vi "Moving_FFID_Analysis.vi"() -> (5 "Plug in titles":string[](array[string]), 7 "Plug in values":string[](array[string]))   [LabVIEW 2010]
uses:
  Globals/Plug_in_data_global.vi
  Globals/Meas_global.vi
  <vilib>/Analysis/NI_AALPro.lvlib
panel:
  in  "Downsize points":i32
  out "Rejected Blocks":i32
  in  "Traverse Speed Factor":string
  in  "Number of Samples":string
  out "Pdf":cluster{"Axis":dbl[], dbl[]}(graph)
  in  "Histogram Time":dbl format="%.2f"
  out "Current Block No":i32
  in  "Save averaged traces?":bool
  out "No of Valid Blocks":dbl
  out "FFID Trace Even":cluster{dbl, dbl, dbl[]}(graph)
  out "FFID Trace odd":cluster{dbl, dbl, dbl[]}(graph)
  out "Source On":i32
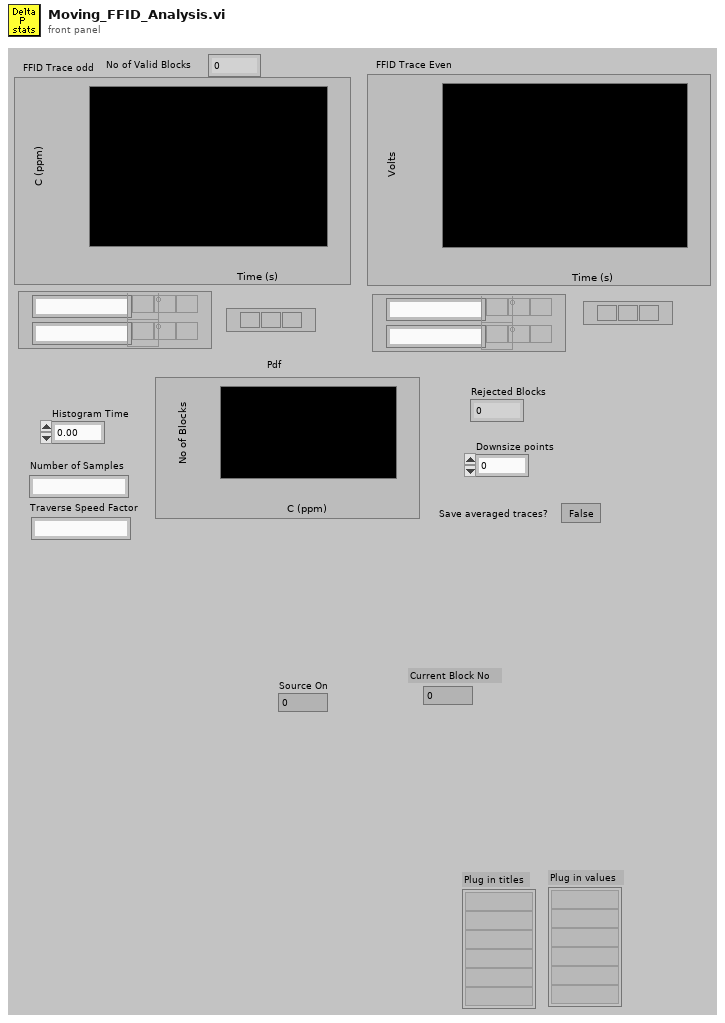
[diagram p1: front panel]
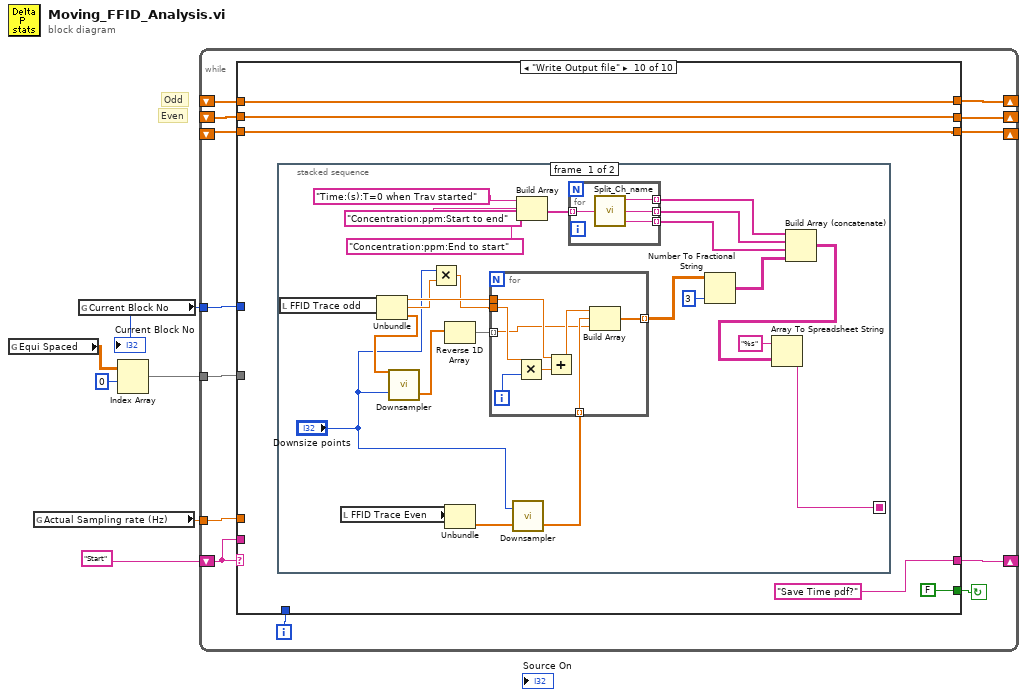
[diagram p0: block diagram]
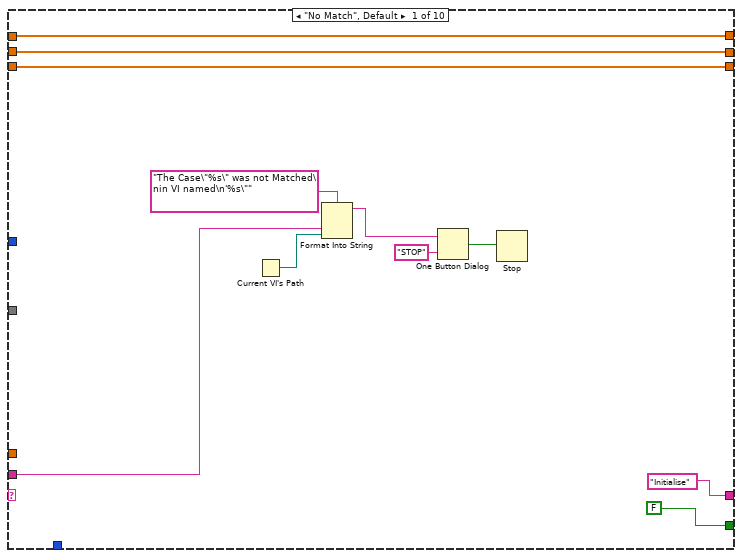
[diagram p2: hidden frame]
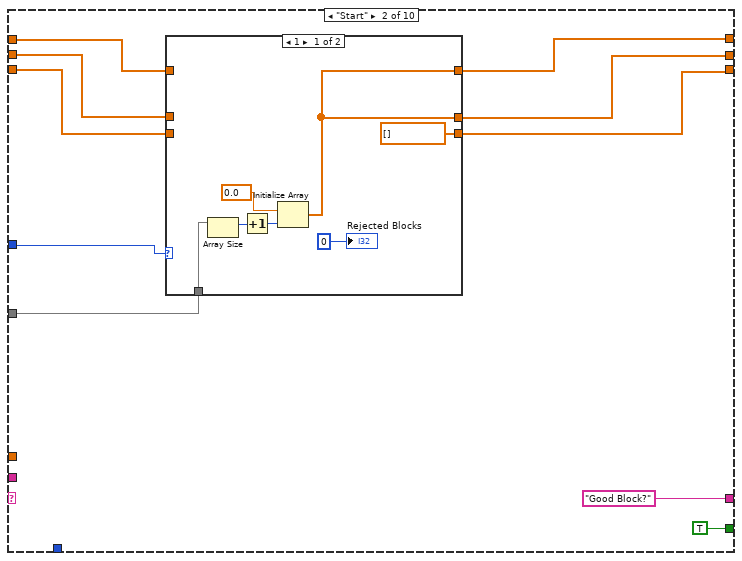
[diagram p3: hidden frame]
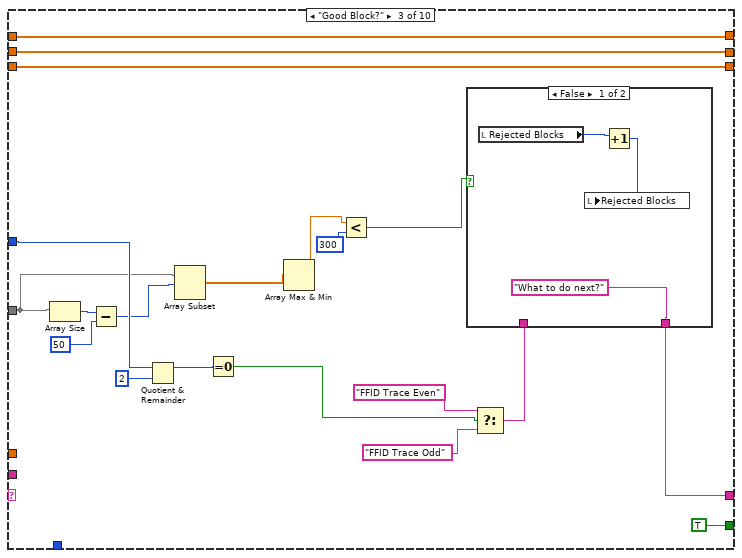
[diagram p5: hidden frame]
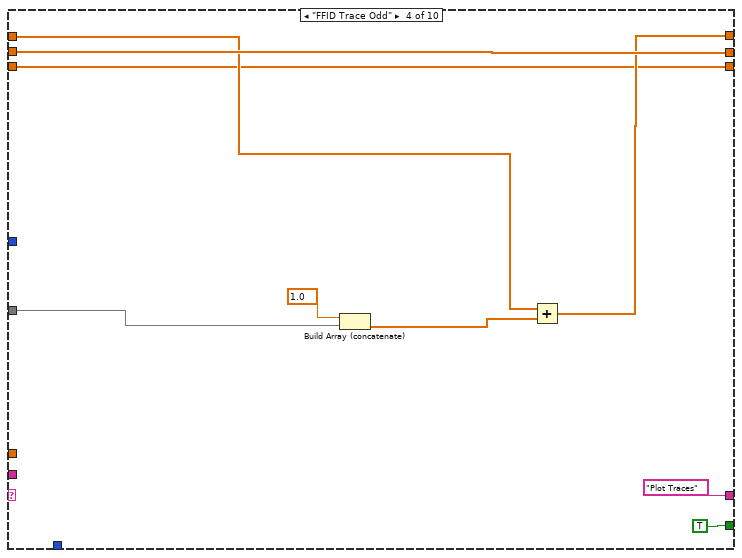
[diagram p7: hidden frame]
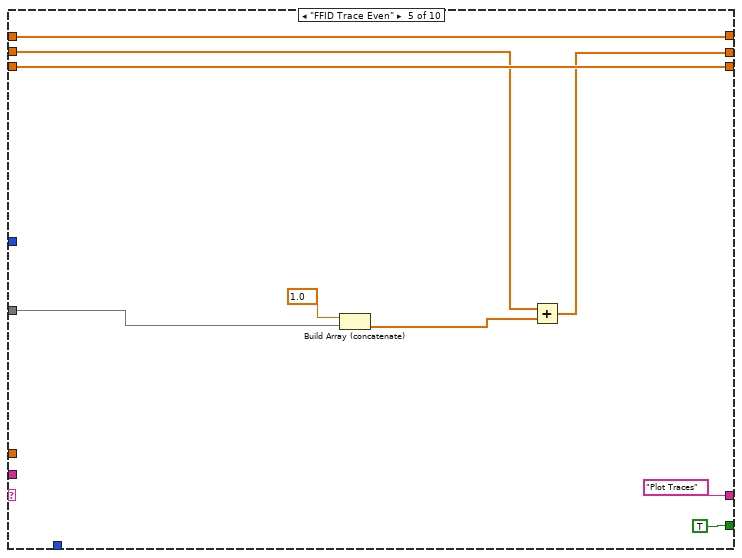
[diagram p8: hidden frame]
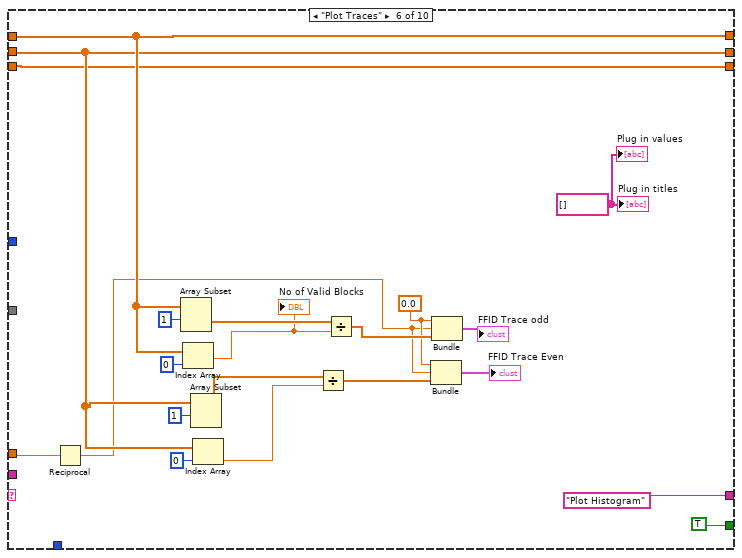
[diagram p9: hidden frame]
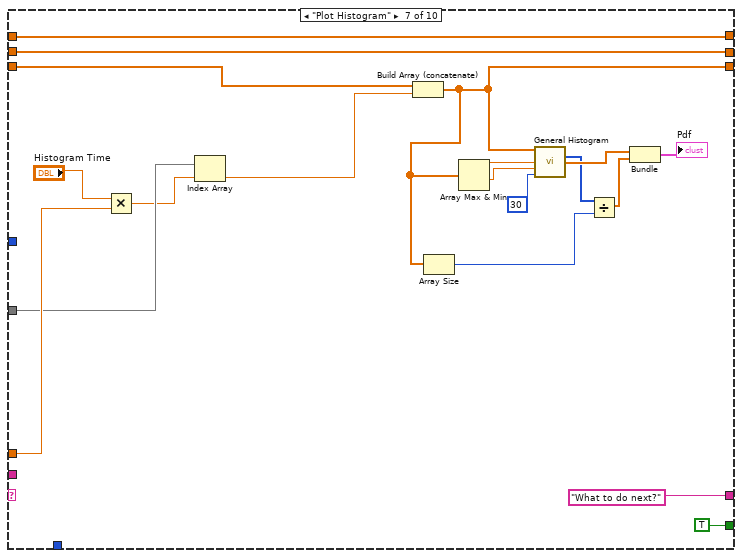
[diagram p10: hidden frame]
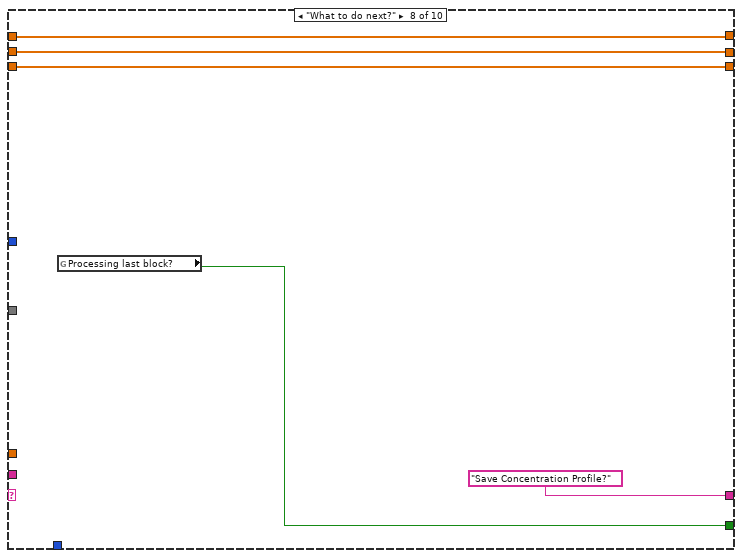
[diagram p11: hidden frame]
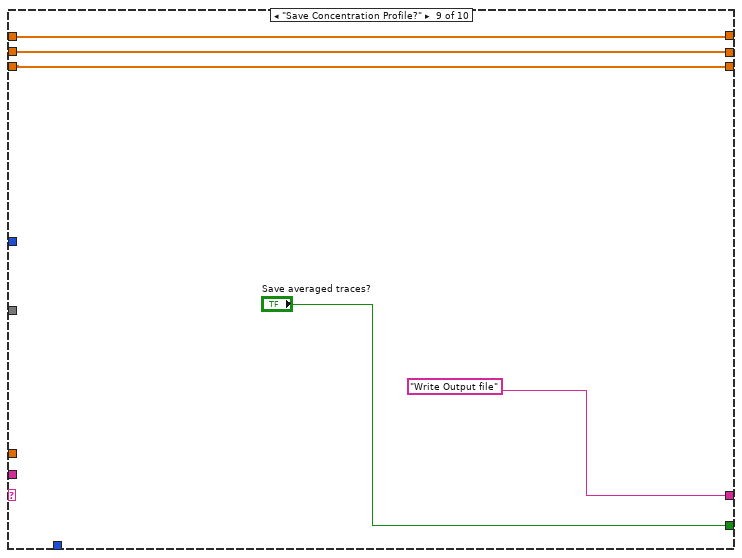
[diagram p12: hidden frame]
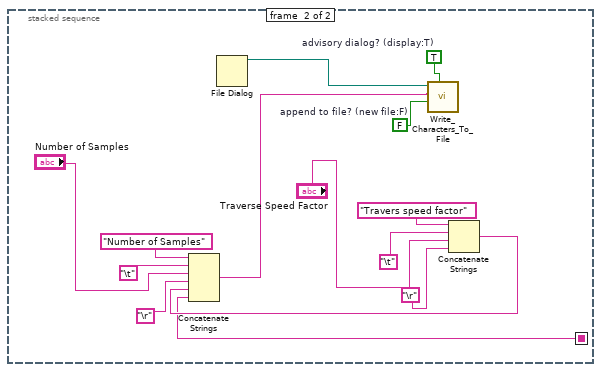
[diagram p13: hidden frame]
diagram:
  # "Even"
  # "Odd"
  n1 = global read "Plug_in_data_global.vi" "Equi Spaced"() -> (w1:dbl[][])
  n2 = global read "Meas_global.vi" "Actual Sampling rate (Hz)"() -> (w3:dbl)
  n3 = global read "Meas_global.vi" "Current Block No"() -> (w2:i32)
  "Current Block No" <- w2
  n4 = Index Array(array=w1, index (row)=0) -> (element=w4:dbl[])  [unwired: 1 in]
  n5 = while {
    shift-left: "Start" -> [w17]
    shift-right: [w18] -> _
    shift-right: [w16] -> _
    shift-left: _ -> [w13]
    shift-right: [w15] -> _
    shift-left: _ -> [w14]
    tunnel: w4 -> [w12]
    tunnel: w3 -> [w11]
    tunnel: w2 -> [w10]
    shift-right: [w7] -> _
    shift-left: _ -> [w8]
    i -> [w9]
    stop <- w19 continue-if-true
    n6 = case shown="\"Write Output file\"" w17 {
      tunnel: [FALSE TRUE ("Processing last block?") TRUE ("Processing last block?") TRUE ("Processing last block?") TRUE ("Processing last block?") TRUE ("Processing last block?") TRUE ("Processing last block?") w133 "Save averaged traces?" FALSE ("Processing last block?")] -> w19
      tunnel: ["Initialise" "Good Block?" w52 "Plot Traces" "Plot Traces" "Plot Histogram" ("f") "What to do next?" ("f") "Save Concentration Profile?" ("t") "Write Output file" "Save Time pdf?"] -> w18
      tunnel: w17 -> [w25 _ _ _ _ _ _ _ _ _]
      tunnel: [w22 w39 w70 w80 w86 w111 w132 w137 w142 w147] -> w16
      tunnel: [w21 w37 w69 w81 w84 w107 w131 w136 w138 w146] -> w15
      tunnel: w14 -> [w21 w36 w69 w81 w85 w107 w131 w136 w138 w146]
      tunnel: w13 -> [w22 w38 w70 w79 w86 w111 w132 w137 w142 w147]
      tunnel: w12 -> [_ w35 w60 w75 w87 _ w128 _ _ _]
      tunnel: w11 -> [_ _ _ _ _ w103 w129 _ _ _]
      tunnel: w10 -> [_ w34 w65 _ _ _ _ _ _ _]
      tunnel: w9 -> [_ _ _ _ _ _ _ _ _ _]
      tunnel: w8 -> [w20 w32 w68 w76 w88 w98 w125 w135 w141 w143]
      tunnel: [w20 w33 w68 w76 w88 w98 w117 w135 w141 w143] -> w7
      frame "No Match", Default {
        n7 = Current VI's Path() -> (path=w24:path)
        n8 = Format Into String(format string="The Case\"%s\" was not Matched\nin VI named\n'%s\"" ("Format String"), w25, w24) -> (resulting string=w28:string)  [unwired: 2 in, 1 out]
        n9 = One Button Dialog(message=w28, button name ("OK")="STOP") -> (true=w26:bool)
        n10 = Stop(stop? (T)=w26) -> ()
      }
      frame "Start" {
        n11 = case shown="1" w34 {
          tunnel: [w44 w50] -> w39
          tunnel: w38 -> [_ w50]
          tunnel: [w44 w49] -> w37
          tunnel: w36 -> [_ w49]
          tunnel: w35 -> [w47 _]
          tunnel: [dbl[] [] w48] -> w33
          tunnel: w32 -> [_ w48]
          frame 1 {
            n12 = Array Size(array=w47) -> (size(s)=w46:i32)
            n13 = Increment(x=w46) -> (x+1=w42:i32)
            n14 = Initialize Array(0.0 ("element"), w42) -> (w44:dbl[])
            "Rejected Blocks" <- 0 ("Rejected Blocks")
          }
          frame 2, Default {
          }
        }
      }
      frame "Good Block?" {
        n15 = Array Size(array=w60) -> (size(s)=w59:i32)
        n16 = Subtract(x=w59, y=50) -> (x-y=w58:i32)
        n17 = Quotient & Remainder(x=w65, y=2) -> (x-y*floor(x/y)=w64:i32)  [unwired: 1 out]
        n18 = Array Subset(array=w60, index=w58) -> (w56:dbl[])  [unwired: 1 in]
        n19 = Equal To 0?(x=w64) -> (x = 0?=w63:bool)
        n20 = Array Max & Min(array=w56) -> (max value=w55:dbl)  [unwired: 3 out]
        n21 = Less?(x=w55, y=300) -> (x < y?=w53:bool)
        n22 = Select(t="FFID Trace Even", s=w63, f="FFID Trace Odd") -> (s? t:f=w51:string)
        n23 = case shown="False" w53 {
          tunnel: ["What to do next?" ("f") w74] -> w52
          tunnel: w51 -> [_ w74]
          frame False {
            n24 = local read "Rejected Blocks"() -> (w72:i32)
            n25 = Increment(x=w72) -> (x+1=w71:i32)
            n26 = local write "Rejected Blocks"(w71) -> ()
          }
          frame True {
          }
        }
      }
      frame "FFID Trace Odd" {
        n27 = Build Array (concatenate)(1.0, w75) -> (w77:dbl[])
        n28 = Add(x=w79, y=w77) -> (x+y=w80:dbl[])
      }
      frame "FFID Trace Even" {
        n29 = Build Array (concatenate)(1.0, w87) -> (w89:dbl[])
        n30 = Add(x=w85, y=w89) -> (x+y=w84:dbl[])
      }
      frame "Plot Traces" {
        w94 = string[] [] ("Plug in titles")
        w97 = 0.0
        n31 = Reciprocal(x=w103) -> (1/x=w93:dbl)
        n32 = Array Subset(array=w111, index=1) -> (w110:dbl[])  [unwired: 1 in]
        n33 = Index Array(array=w111, index=0) -> (element=w95:dbl)
        "No of Valid Blocks" <- w95
        n34 = Array Subset(array=w107, index=1) -> (w106:dbl[])  [unwired: 1 in]
        n35 = Index Array(array=w107, index=0) -> (element=w105:dbl)
        n36 = Divide(x=w106, y=w105) -> (x/y=w101:dbl[])
        n37 = Divide(x=w110, y=w95) -> (x/y=w99:dbl[])
        n38 = Bundle(w97, w93, w101) -> (→"FFID Trace Even":cluster{dbl, dbl, dbl[]})  [unwired: 1 out]
        n39 = Bundle(w97, w93, w99) -> (→"FFID Trace odd":cluster{dbl, dbl, dbl[]})  [unwired: 1 out]
        "Plug in values" <- w94
        "Plug in titles" <- w94
      }
      frame "Plot Histogram" {
        n40 = Multiply(x="Histogram Time", y=w129) -> (x*y=w127:dbl)
        n41 = Index Array(array=w128, index=w127) -> (element=w126:dbl)
        n42 = Build Array (concatenate)(w125, w126) -> (w117:dbl[])
        n43 = Array Size(array=w117) -> (size(s)=w115:i32)
        n44 = Array Max & Min(array=w117) -> (max value=w124:dbl, min value=w123:dbl)  [unwired: 2 out]
        n45 = call <vilib>:"General Histogram.vi"("X"=w117, "max"=w124, "min"=w123, "# bins"=30) -> ("Histogram"=w116:i32[], "Axis"=w121:dbl[])  [unwired: 2 in, 8 out]
        n46 = Divide(x=w116, y=w115) -> (x/y=w114:dbl[])
        n47 = Bundle("Axis"=w121, w114) -> (→"Pdf":cluster{"Axis":dbl[], dbl[]})  [unwired: 1 out]
      }
      frame "What to do next?" {
        n48 = global read "Meas_global.vi" "Processing last block?"() -> (w133:bool)
      }
      frame "Save Concentration Profile?" {
      }
      frame "Write Output file" {
        n49 = stacked-sequence {
          seq-local: [w163 _] -> [_ w184]
          frame #0 {
            n50 = local read "FFID Trace odd"() -> (w171:cluster{dbl, dbl, dbl[]})
            n51 = local read "FFID Trace Even"() -> (w162:cluster{dbl, dbl, dbl[]})
            n52 = Unbundle(w171) -> (w170:dbl, w150:dbl, w154:dbl[])
            n53 = call "Downsampler.vi"("Input Array"=w154, "Averaging samples"="Downsize points") -> ("Downsampled Array"=w153:dbl[])  [unwired: 1 out]
            n54 = Multiply(x="Downsize points", y=w150) -> (x*y=w148:dbl)
            n55 = Reverse 1D Array(array=w153) -> (reversed array=w155:dbl[])
            n56 = Unbundle(w162) -> (w152:dbl[])  [unwired: 2 out]
            n57 = call "Downsampler.vi"("Input Array"=w152, "Averaging samples"="Downsize points") -> ("Downsampled Array"=w151:dbl[])  [unwired: 1 out]
            n58 = for {
              tunnel: w148 -> [w182]
              tunnel: w170 -> [w181]
              tunnel: w155 -> [w176] mode=indexing
              tunnel: [w179] -> w168 mode=indexing
              tunnel: w151 -> [w177] mode=indexing
              i -> [w183]
              n59 = Multiply(x=w182, y=w183) -> (x*y=w180:dbl)
              n60 = Add(x=w181, y=w180) -> (x+y=w178:dbl)
              n61 = Build Array(w178, w177, w176) -> (w179:dbl[])
            }
            n62 = Build Array("Time:(s):T=0 when Trav started", "Concentration:ppm:Start to end", "Concentration:ppm:End to start") -> (w159:string[])
            n63 = for {
              tunnel: w159 -> [w175] mode=indexing
              tunnel: [w174] -> w158 mode=indexing
              tunnel: [w173] -> w157 mode=indexing
              tunnel: [w172] -> w156 mode=indexing
              n64 = call "Split_Ch_name.vi"("Ch name"=w175) -> ("Top level"=w174:string, "Middle"=w173:string, "Low level"=w172:string)
            }
            n65 = Number To Fractional String(number=w168, precision (6)=i16 3) -> (F-format string=w167:string[][])  [unwired: 2 out]
            n66 = Build Array (concatenate)(w158, w157, w156, w167) -> (w165:string[][])
            n67 = Array To Spreadsheet String(array=w165, 3:"%s" ("format string")) -> (spreadsheet string=w163:string)  [unwired: 1 out]
          }
          frame #1 {
            w196 = FALSE  # append to file? (new file:F)
            w197 = TRUE  # advisory dialog? (display:T)
            n68 = File Dialog() -> (3:w186:path)  [unwired: 1 in, 9 out]
            n69 = Concatenate Strings("Travers speed factor", "\t", "Traverse Speed Factor", "\r") -> (w185:string)
            n70 = Concatenate Strings("Number of Samples", "\t", "Number of Samples", "\r", w185, w184) -> (w191:string)
            n71 = call "Write_Characters_To_File.vi"("file path (dialog if empty)"=w186, "advisory dialog? (display:T)"=w197, "character string"=w191, "append to file? (new file:F)"=w196) -> ()  [unwired: 1 in, 4 out]
          }
        }
      }
    }
  }
